vi "01_Main.vi"() -> ()   [LabVIEW 2023]
doc: "This VI shows how to setup and execute a measurement without any user input."
panel:
  out "N":i32=-1
  out "size(s)":i32[](array[numeric])
  in  "Fahrprofil Datei":path
  out "IP-Adresse Antrieb":string="192.168.10.5"
  in  "BETRIEBSART ANTRIEB":bool
  out "Digital Antrieb":dbl
  out "Drehmoment Antrieb":dbl
  out "Status/Fehler Antrieb":dbl
  out "Istgeschwindigkeit Antrieb":dbl
  in  "Digital Antrieb":dbl
  in  "Deceleration Antrieb":dbl
  in  "Acceleration Antrieb":dbl
  in  "Speed Antrieb":dbl
  out "IP-Adresse Last":string
  out "Digital":dbl
  out "Drehmoment":dbl
  out "Status/Fehler":dbl
  out "Istgeschwindigkeit":dbl
  in  "Digital A":dbl
  in  "Deceleration":dbl
  in  "Acceleration":dbl
  in  "Speed":dbl
  out "Reserviert":bool
  out "SWES inaktiv":bool
  out "Geschwindigkeit erreicht":bool
  out "Warnung":bool
  out "Fehler":bool
  out "in Position":bool
  out "Relativposition übernommen":bool
  out "Motor dreht":bool
  out "Bremse geöffnet":bool
  out "Endstufenfreigabe":bool
  out "STO inaktiv":bool
  out "Betriebsbereit":bool
  out "Reserviert 8":bool
  out "SWES inaktiv 2":bool
  out "Geschwindigkeit erreicht 2":bool
  out "Warnung 2":bool
  out "Fehler 2":bool
  out "in Position 2":bool
  out "Relativposition übernommen 2":bool
  out "Motor dreht 2":bool
  out "Bremse geöffnet 2":bool
  out "Endstufenfreigabe 2":bool
  out "STO inaktiv 2":bool
  out "Betriebsbereit 2":bool
  in  "Reserviert 9":bool
  in  "Reservier 2":bool
  in  "Reserviert 10":bool
  in  "Reserviert 11":bool
  in  "Reserviert 12":bool
  in  "Reserviert 13":bool
  in  "Reserviert 14":bool
  in  "Reserviert 2":bool
  in  "Reservier":bool
  in  "Reserviert 3":bool
  in  "Reserviert 4":bool
  in  "Reserviert 5":bool
  in  "Reserviert 6":bool
  in  "Reserviert 7":bool
  in  "Bedienelemente - Lastmotor":enum32{"Standard", "Versteckt"}(tab)
  in  "Enable/EmergencyStop Antrieb":bool
  in  "Fehler_Reset Antrieb":bool
  in  "Antriebsmotor Start":bool
  in  "Enable/ApplicationStop Antrieb":bool=TRUE
  in  "Inhibit L":bool
  in  "Standby Antrieb":bool
  in  "Handshake Antrieb":bool
  in  "AS2 aktivieren Antrieb":bool
  in  "Bremse öffnen Antrieb":bool
  out "Standby aktiv 2":bool
  out "AS2 aktiv 2":bool
  out "Handshake 3":bool
  out "referenziert 2":bool
  in  "Bedienelemente - Antriebsmotor":enum32{"Standard", "Versteckt"}(tab)
  in  "Enable/EmergencyStop":bool
  in  "Enable/ApplicationStop":bool=TRUE
  in  "Fehler_Reset":bool
  in  "Lastmotor Start":bool
  in  "Inhibit":bool
  in  "Standby":bool
  in  "Handshake 2":bool
  in  "AS2 aktivieren":bool
  in  "Bremse öffnen":bool
  out "AS2 aktiv":bool
  out "Handshake":bool
  out "Standby aktiv":bool
  out "referenziert":bool
  out "Numeric":i32
  out "VI wird beendet":string
  in  "VI-Stopp":bool
  out "Diagram 2":waveform(dbl)(graph)
  in  "Kanal 2":i32=2 min=1 max=4 step=1
  in  "Kanal":i32=1 min=1 max=4 step=1
  in  "Datei-Pfad":path
  out "Diagram":waveform(dbl)(graph)
  in  "Messung":bool=TRUE
  out "HBM Driver\nLicense is valid":bool
  # "Im Handbetrieb im Feld \"Speed\" die Soll-Geschwindigkeit vorgeben. Nach Betätigung des Start-Knopfes läuft der Motor an. \n\nFür den Antrieb ist das Laden von Fahrprofilen möglich. Dazu Fahrprofil Datei auswählen, START-Knopf drücken und dann BETRIEBSART ANTRIEB auf \"Fahrprofile laden\" schalten."
  # "Handbetrieb"
  # "Fahrprofil laden"
  # "Manuelle Ansteuerung des Last-Motors"
  # "Manuelle Ansteuerung des Antrieb-Motors"
  # "Datenaquise mit dem HBM Messverstärker"
  # "Messung mit START starten.\n\nWenn die Messdaten gespeichert werden sollen, muss vor \ndem Starten der Messung ein gültiger Dateipfad angegeben werden."
  # "Datenaufzeichnung"
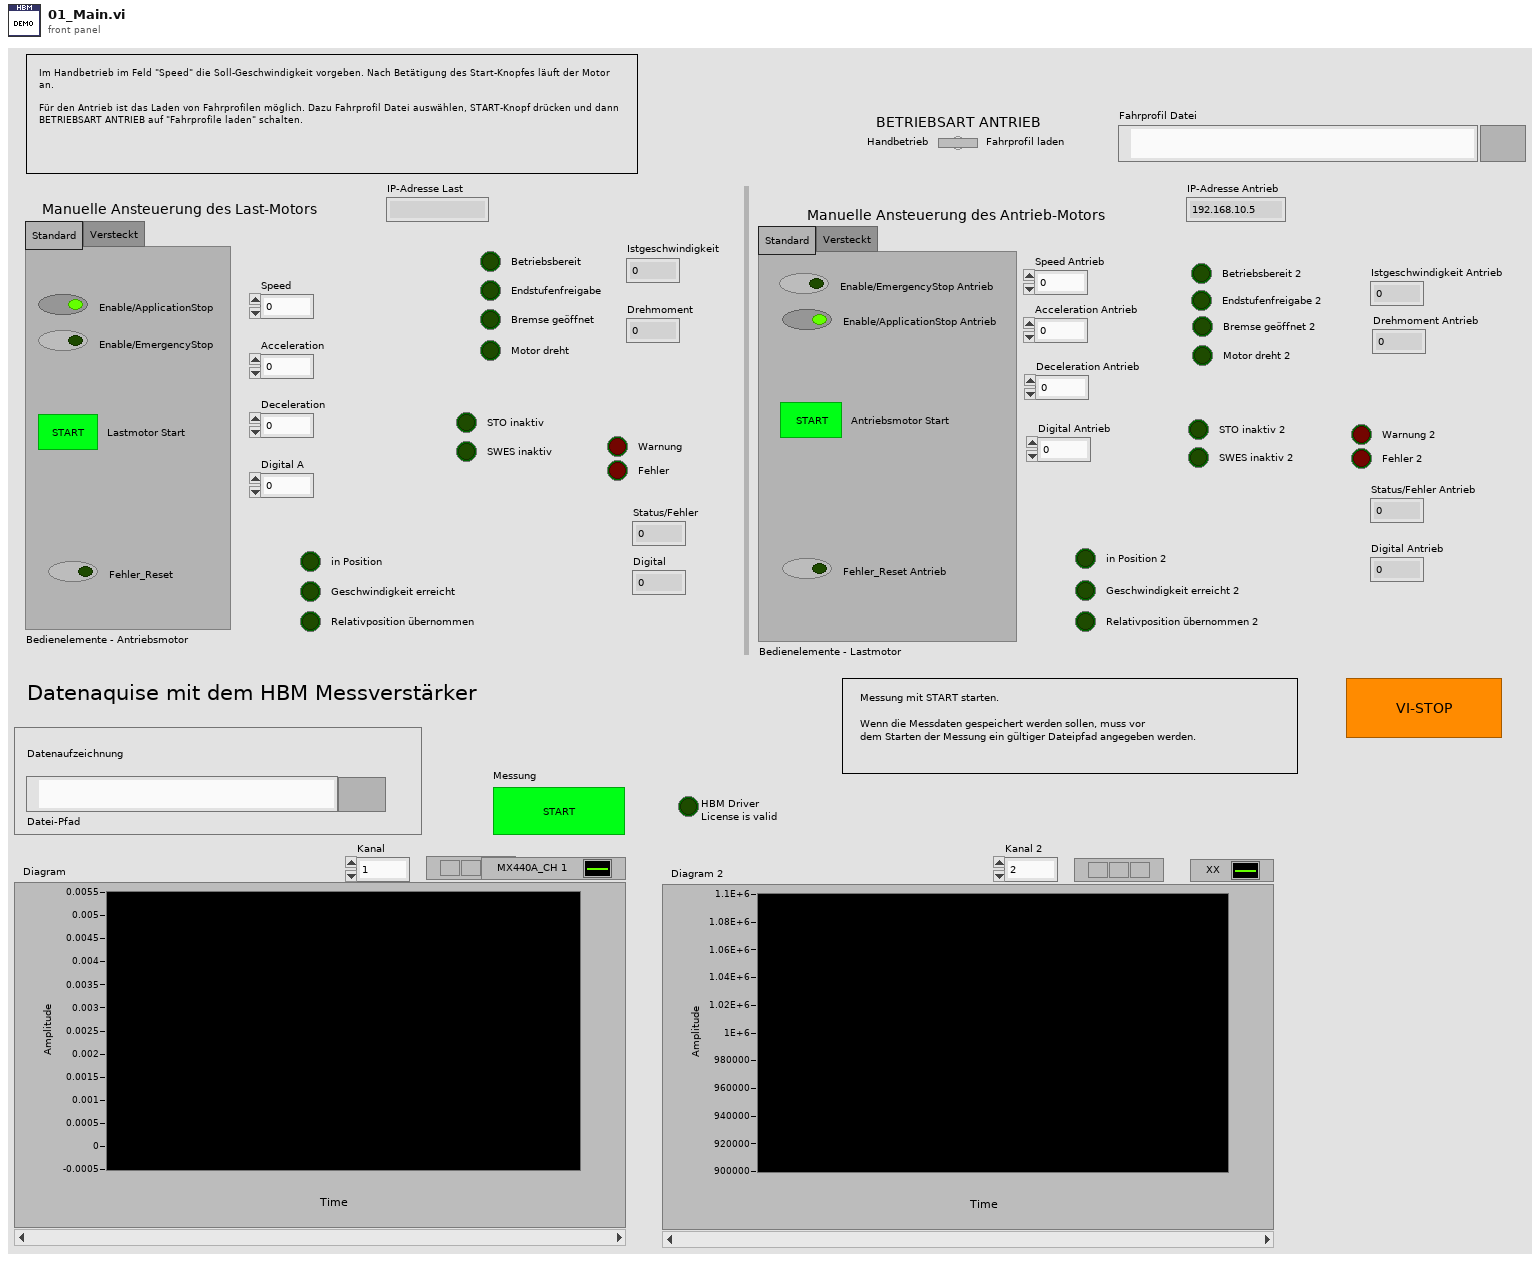
[diagram p1: front panel]
types:
  T1 = cluster{"Devices":refnum<k24>[], "Signals":refnum<k24>[]}
  T2 = enum16{"open", "replace", "create", "open or create", "replace or create", "replace or create with confirmation"}
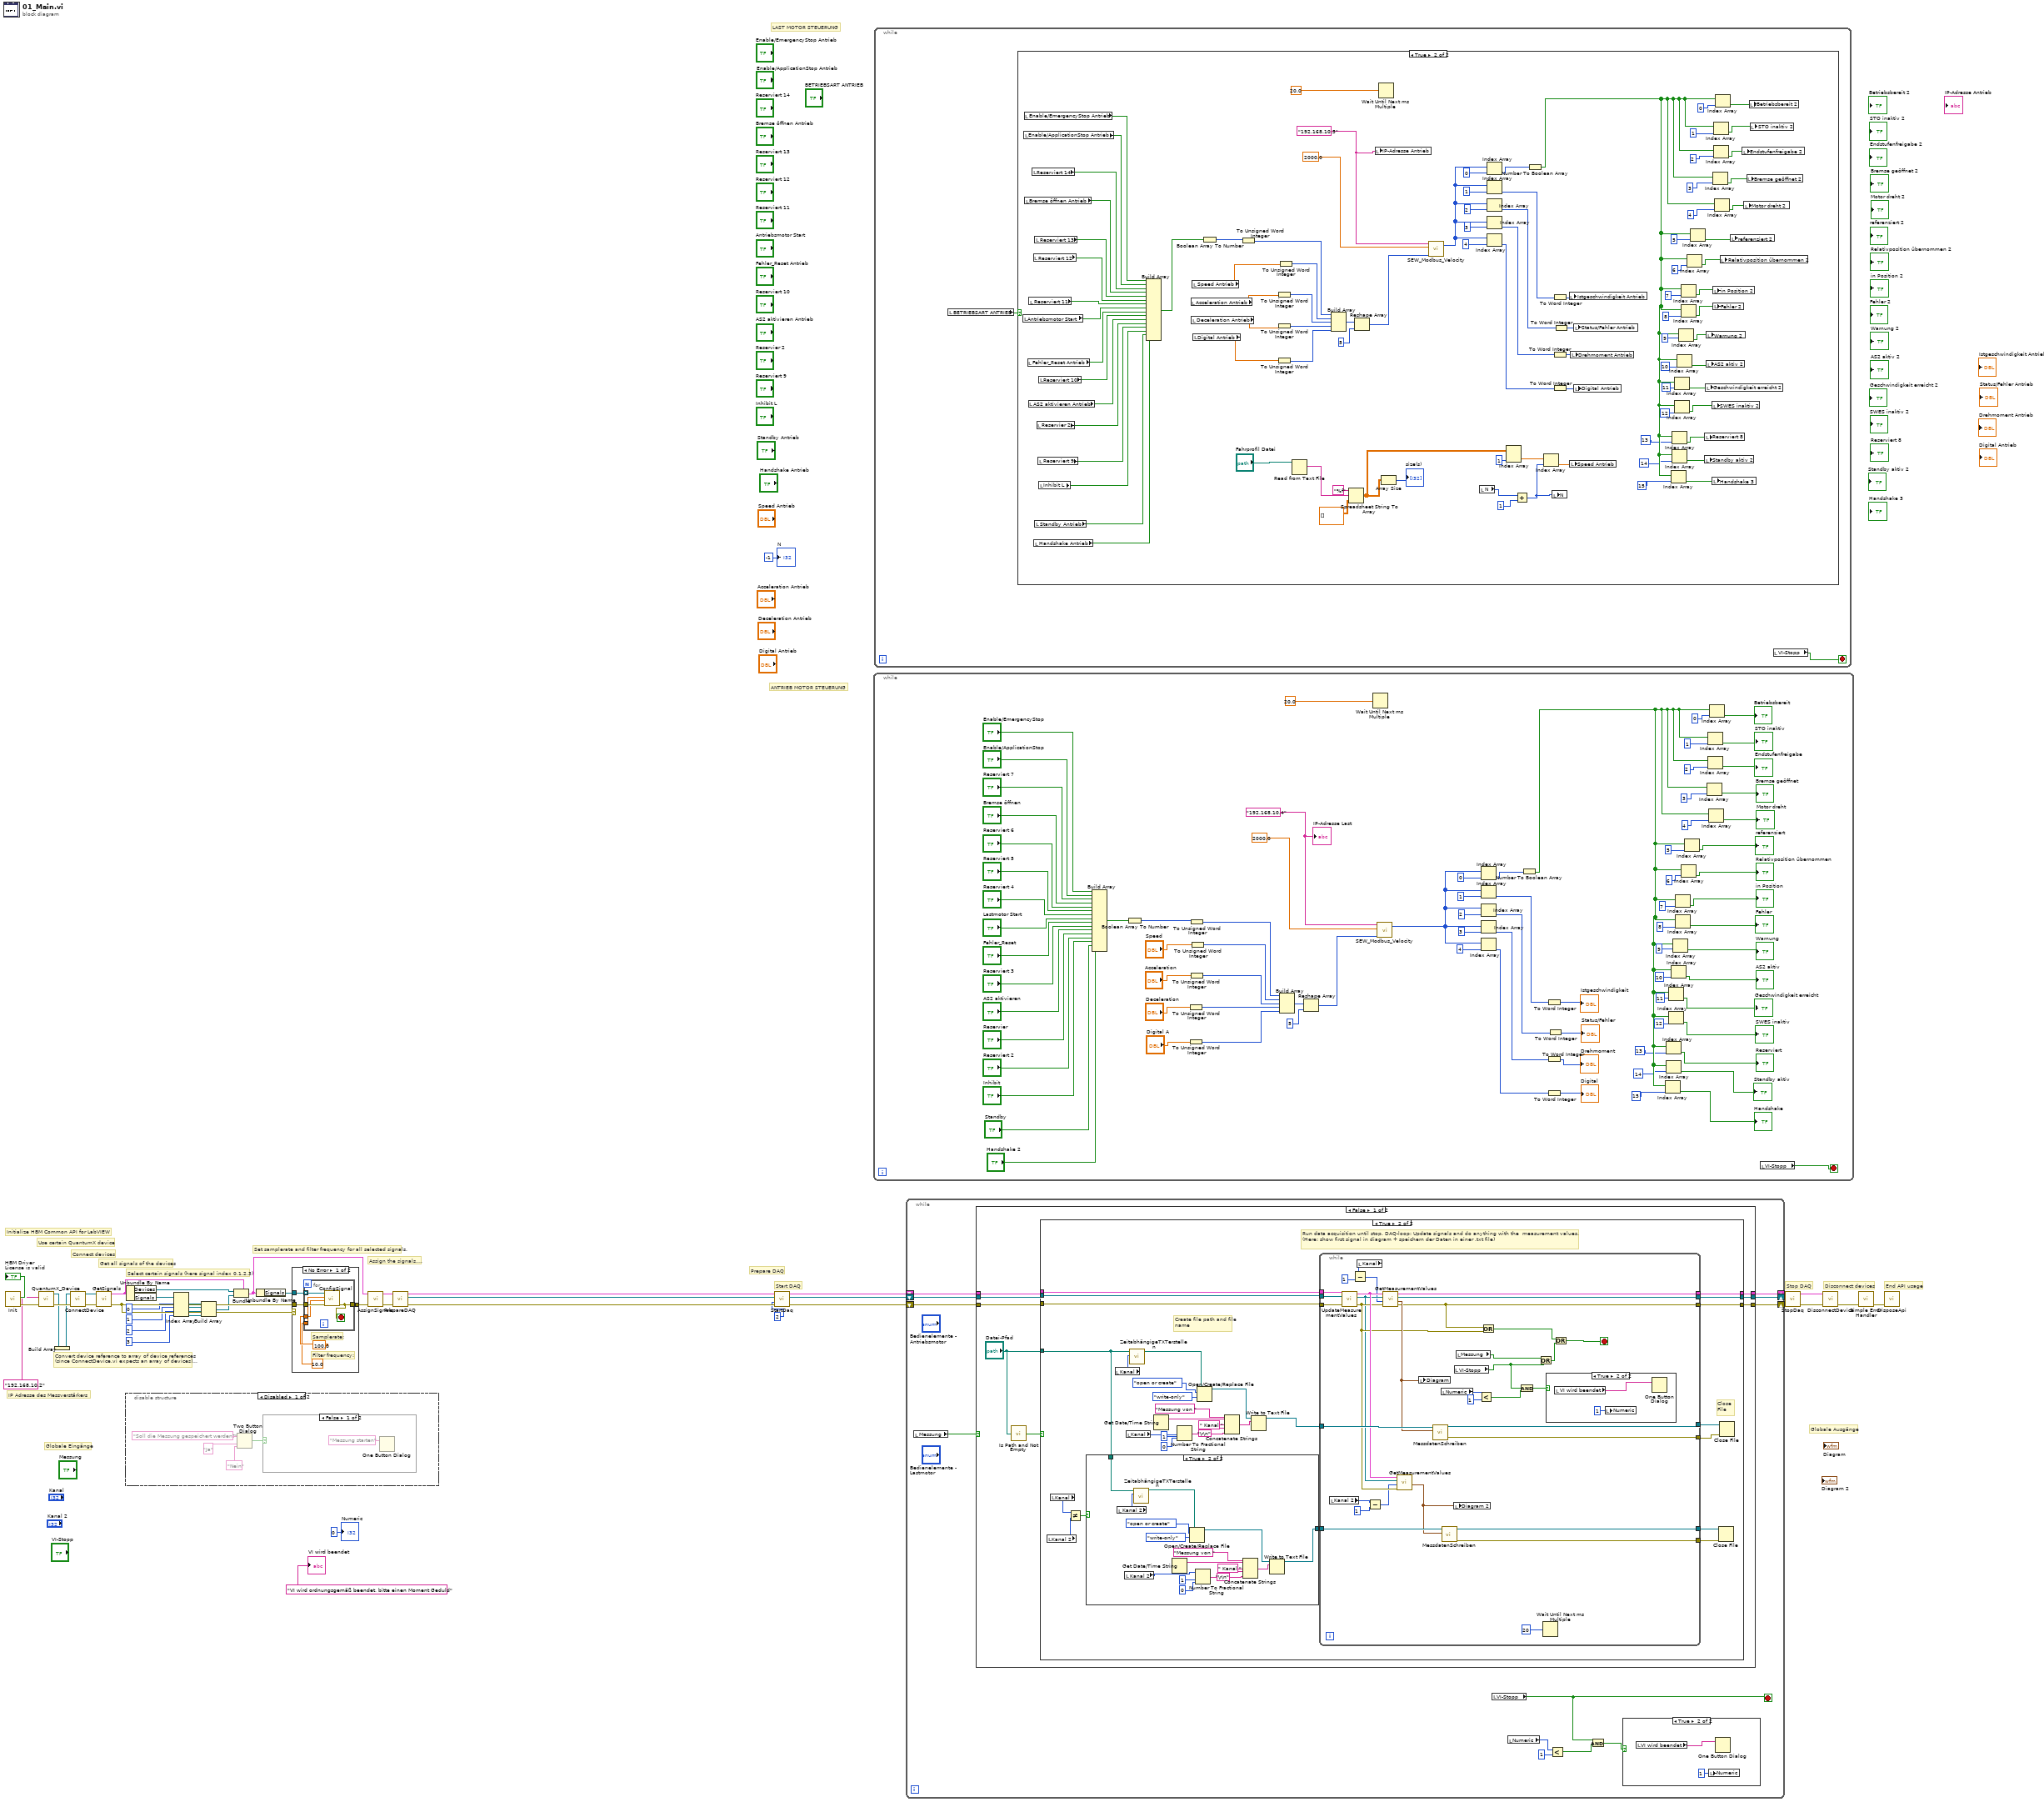
[diagram p0: block diagram]
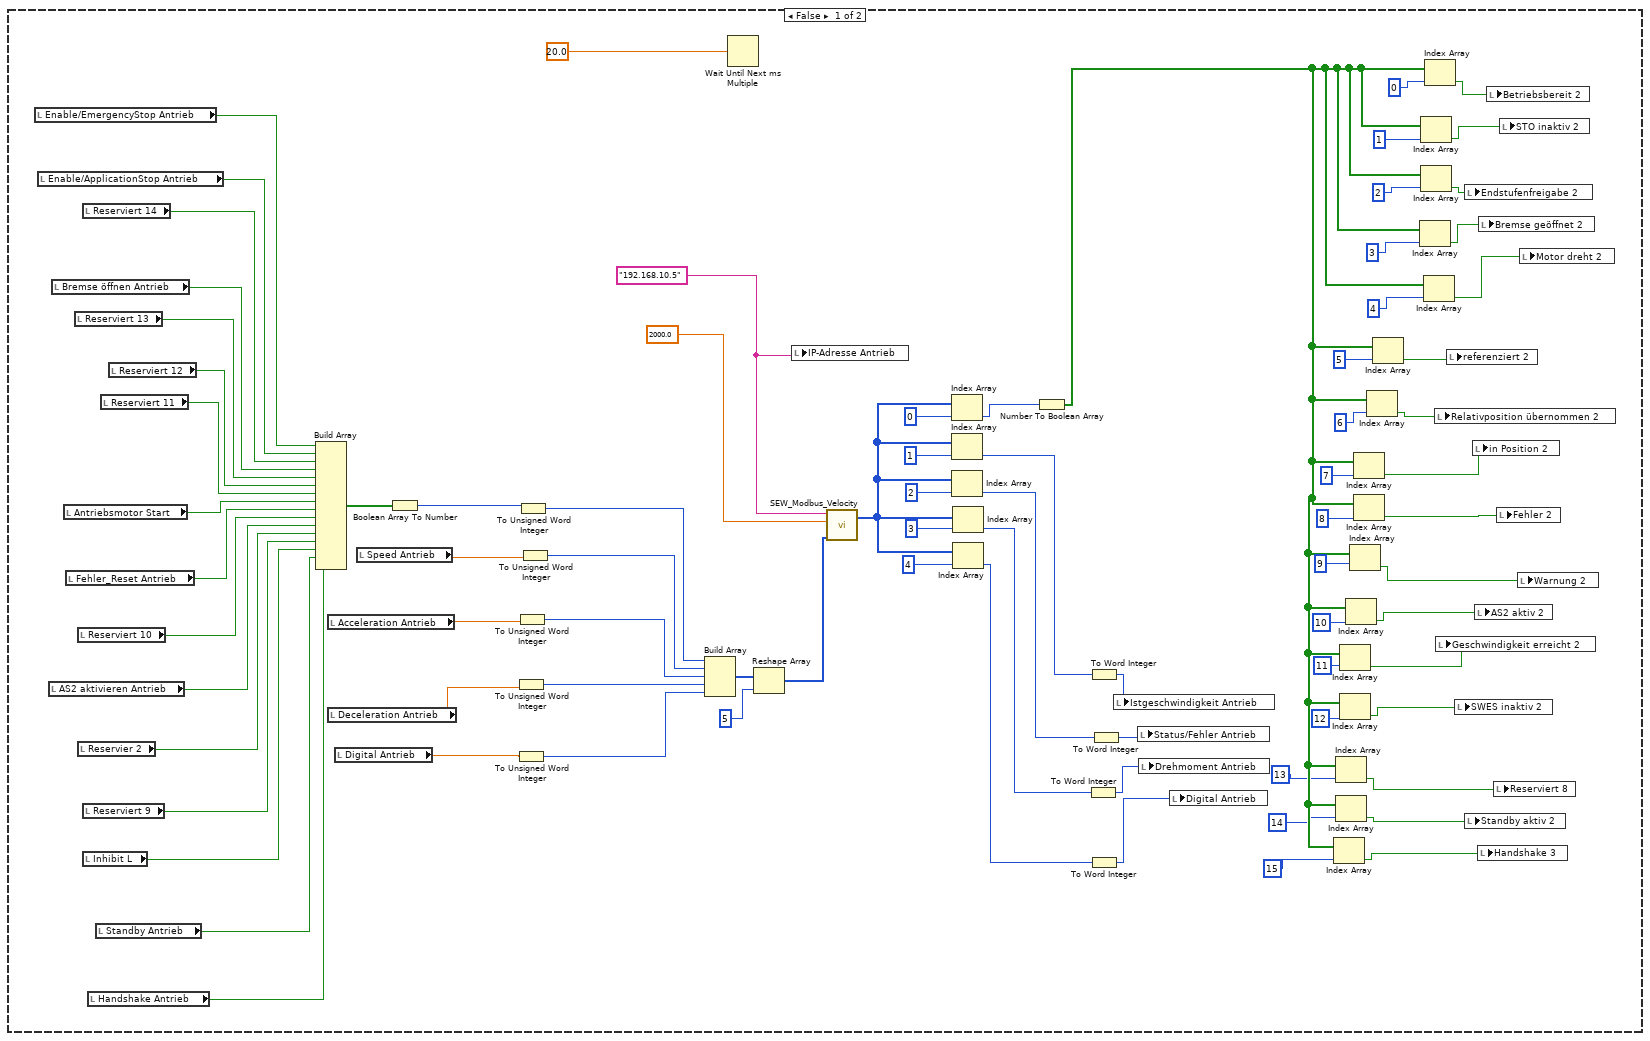
[diagram p2: hidden frame]
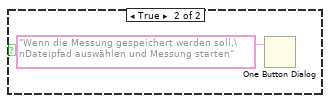
[diagram p3: hidden frame]
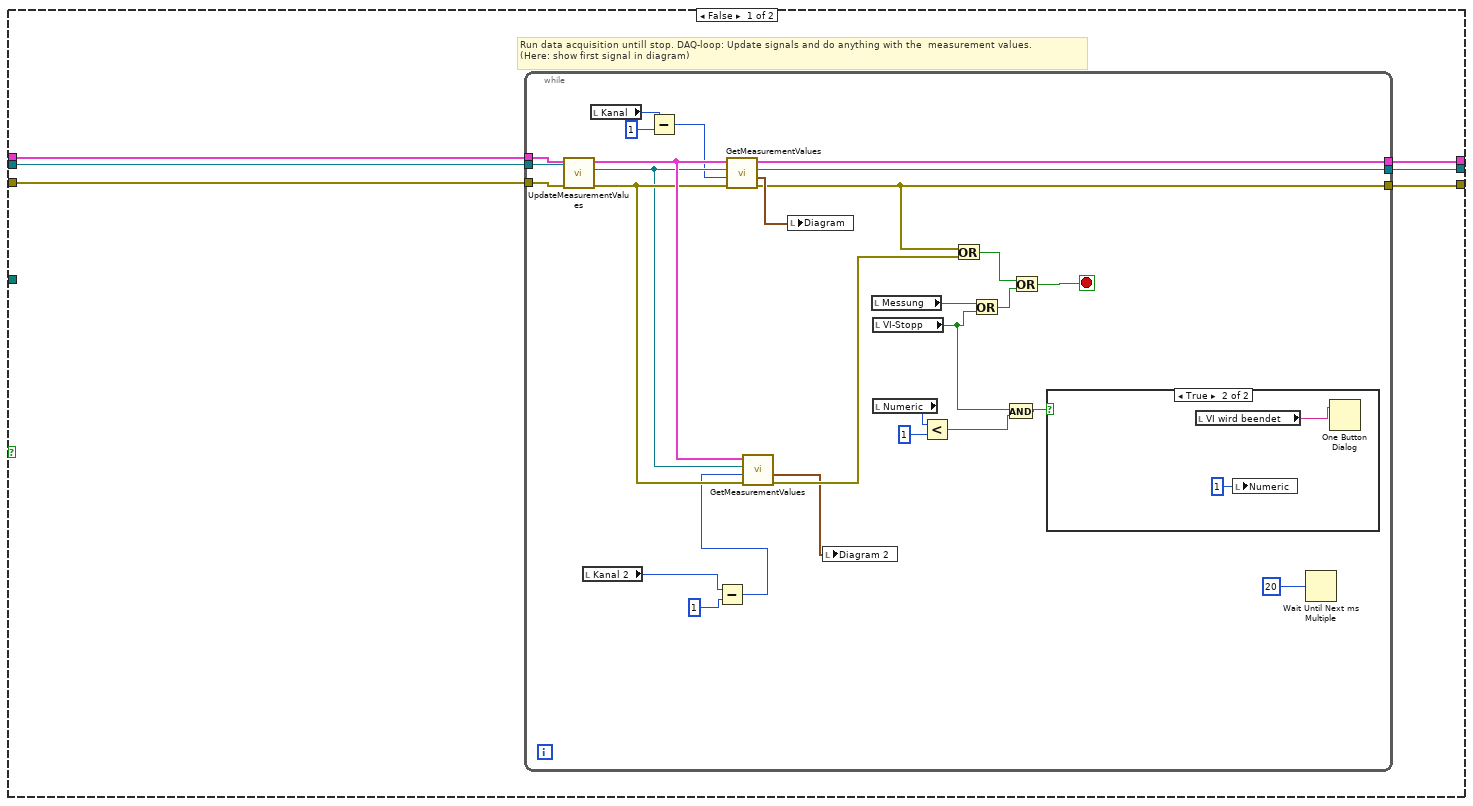
[diagram p6: hidden frame]
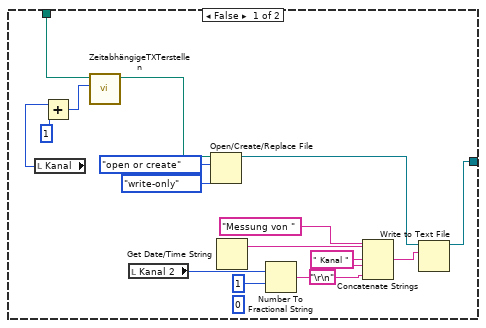
[diagram p8: hidden frame]
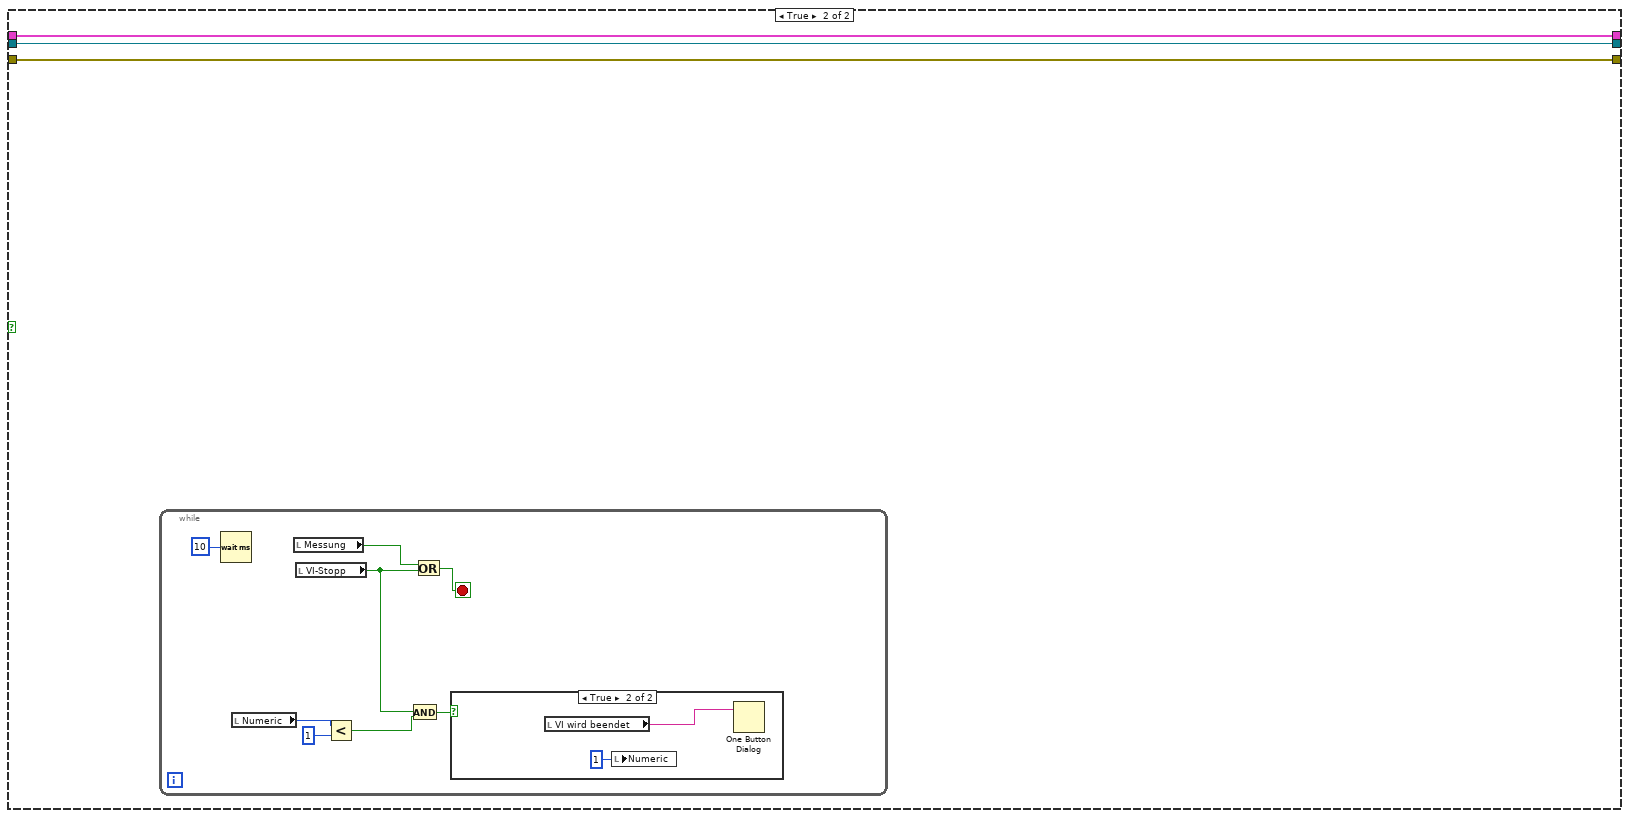
[diagram p10: hidden frame]
diagram:
  # "ANTRIEB MOTOR STEUERUNG"
  # "LAST MOTOR STEUERUNG"
  # "Globale Ausgänge"
  # "Globale Eingänge"
  # "IP Adresse des Messverstärkers"
  # "Convert device reference to array of device references\n(since ConnectDevice.vi expects an array of devices)..."
  # "Disconnect devices"
  # "Set samplerate and filter frequency for all selected signals."
  # "Initialize HBM Common API for LabVIEW"
  # "End API usage"
  # "Stop DAQ"
  # "Start DAQ"
  # "Prepare DAQ"
  # "Select certain signals (here signal index 0,1,2,3)"
  # "Get all signals of the devices"
  # "Connect devices"
  # "Use certain QuantumX device"
  # "Assign the signals...."
  n1 = call <userlib>:"Init.vi"() -> ("LicenseIsValid"=→"HBM Driver\nLicense is valid":bool, "Error out"=w13:errorcluster)  [unwired: 8 in, 1 out]
  n2 = call <userlib>:"QuantumX_Device.vi"("Error in"=w13, "IPAddress"="192.168.10.2" ("IPAddress of QuantumX device")) -> ("Error out"=w14:errorcluster, "Device"=w11:refnum<k24>)  [unwired: 6 in]
  n3 = Build Array(w11) -> (w10:refnum<k24>[])
  n4 = call <userlib>:"ConnectDevice.vi"("Error in"=w14, "Devices"=w10) -> ("Error out"=w36:errorcluster, "Devices"=w35:refnum<k24>[])  [unwired: 7 in, 1 out]
  n5 = call <userlib>:"GetSignals.vi"("Error in"=w36, "Devices"=w35) -> ("Error out"=w30:errorcluster, "DevicesAndSignals"=w31:T1)  [unwired: 8 in]
  n6 = disable-structure shown="Disabled" {
    frame Disabled {
      n7 = Two Button Dialog(message="Soll die Messung gespeichert werden?", 1:"Nein" ("F button name (\"Cancel\")"), 2:"Ja" ("T button name (\"OK\")")) -> (T button?=w47:bool)
      n8 = case shown="False" w47 {
        frame False {
          n9 = One Button Dialog(message="Messung starten") -> ()  [unwired: 1 in, 1 out]
        }
        frame True {
          n10 = One Button Dialog(message="Wenn die Messung gespeichert werden soll,\nDateipfad auswählen und Messung starten") -> ()  [unwired: 1 in, 1 out]
        }
      }
    }
    frame Enabled {
    }
  }
  n11 = Unbundle By Name(w31) -> ("Devices"=w24:refnum<k24>[], "Signals"=w28:refnum<k24>[])
  n12 = Index Array(array=w28, index #1=0 ("Index"), index #2=1 ("Index"), index #3=2 ("Index"), index #4=3 ("Index")) -> (element #1=w27:refnum<k24>, element #2=w26:refnum<k24>, element #3=w19:refnum<k24>, element #4=w18:refnum<k24>)
  n13 = Build Array(w27, w26, w19, w18) -> (w25:refnum<k24>[])
  n14 = Bundle(cluster=w31, "Devices"=w24, "Signals"=w25) -> (w32:T1)
  n15 = Unbundle By Name(w32) -> ("Signals"=w43:refnum<k24>[])
  n16 = case shown="No Error" w30 {
    tunnel: w30 -> [w54 w60]
    tunnel: w43 -> [w53 _]
    tunnel: [w52 w60] -> w42
    frame No Error {
      # "Filter frequency:"
      # "Samplerate:"
      n17 = for {
        tunnel: w54 -> [w59]
        tunnel: 100.0 ("SampleRate") -> [w58]
        tunnel: 10.0 ("FilterFrequency") -> [w57]
        tunnel: w53 -> [w56] mode=indexing
        tunnel: [w55] -> w52
        stop <- w55 stop-if-true
        n18 = call <userlib>:"ConfigSignal.vi"("Error in"=w59, "SampleRate"=w58, "FilterFrequency"=w57, "Signal"=w56) -> ("Error out"=w55:errorcluster)  [unwired: 7 in]
      }
    }
    frame Error {
    }
  }
  n19 = call <userlib>:"AssignSignals.vi"("Error in"=w42, "DevicesAndSignals"=w32) -> ("Error out"=w40:errorcluster, "DevicesAndSignals"=w41:T1)  [unwired: 8 in]
  n20 = call <userlib>:"PrepareDAQ.vi"("Error in"=w40, "DevicesAndSignals"=w41) -> ("Error out"=w37:errorcluster, "DaqMeasurement"=w38:refnum<k24>, "DevicesAndSignals"=w39:T1)  [unwired: 7 in]
  n21 = call <userlib>:"StartDaq.vi"("DevicesAndSignals"=w39, "DaqMeasurement"=w38, "AcquisitionMode"=2, "Error in"=w37) -> ("DevicesAndSignals"=w6:T1, "DaqMeasurement"=w5:refnum<k24>, "Error out"=w4:errorcluster)  [unwired: 7 in, 2 out]
  n22 = while {
    stop <- w102 stop-if-true
    w101 = "192.168.10.4"
    n23 = Build Array("Enable/EmergencyStop", "Enable/ApplicationStop", "Reserviert 7", "Bremse öffnen", "Reserviert 6", "Reserviert 5", "Reserviert 4", "Lastmotor Start", "Fehler_Reset", "Reserviert 3", "AS2 aktivieren", "Reservier", "Reserviert 2", "Inhibit", "Standby", "Handshake 2") -> (w135:bool[])
    n24 = Boolean Array To Number(Boolean array=w135) -> (number=w136:u32)
    n25 = To Unsigned Word Integer(number="Deceleration") -> (unsigned 16bit integer=w139:u16)
    n26 = To Unsigned Word Integer(number="Digital A") -> (unsigned 16bit integer=w140:u16)
    n27 = To Unsigned Word Integer(number="Acceleration") -> (unsigned 16bit integer=w138:u16)
    n28 = To Unsigned Word Integer(number=w136) -> (unsigned 16bit integer=w137:u16)
    n29 = To Unsigned Word Integer(number="Speed") -> (unsigned 16bit integer=w141:u16)
    n30 = Build Array(w137, w141, w138, w139, w140) -> (w142:u16[])
    n31 = Reshape Array(w142, 5) -> (w132:u16[])
    n32 = Wait Until Next ms Multiple(millisecond multiple=20.0 ("Update(ms)")) -> ()  [unwired: 1 out]
    n33 = call "SEW_Modbus_Velocity.vi"("Remote IP Address"=w101, "Timeout [ms]"=2000.0 ("Timeout (ms)"), "Output (Write Multiple Register) 2"=w132) -> ("Input (Read Holding Register) 2"=w130:u16[])  [unwired: 3 in]
    n34 = Index Array(array=w130, index=0) -> (element=w120:u16)
    n35 = Index Array(array=w130, index=1) -> (element=w121:u16)
    n36 = Index Array(array=w130, index=2) -> (element=w122:u16)
    n37 = Index Array(array=w130, index=3) -> (element=w123:u16)
    n38 = Index Array(array=w130, index=4) -> (element=w124:u16)
    n39 = Number To Boolean Array(number=w120) -> (Boolean array=w119:bool[])
    n40 = To Word Integer(number=w123) -> (16bit integer=→"Drehmoment":i16)
    n41 = To Word Integer(number=w121) -> (16bit integer=→"Istgeschwindigkeit":i16)
    n42 = To Word Integer(number=w124) -> (16bit integer=→"Digital":i16)
    n43 = To Word Integer(number=w122) -> (16bit integer=→"Status/Fehler":i16)
    n44 = Index Array(array=w119, index=15) -> (element=→"Handshake":bool)
    n45 = Index Array(array=w119, index=13) -> (element=→"Reserviert":bool)
    n46 = Index Array(array=w119, index=14) -> (element=→"Standby aktiv":bool)
    n47 = Index Array(array=w119, index=11) -> (element=→"Geschwindigkeit erreicht":bool)
    n48 = Index Array(array=w119, index=12) -> (element=→"SWES inaktiv":bool)
    n49 = Index Array(array=w119, index=10) -> (element=→"AS2 aktiv":bool)
    n50 = Index Array(array=w119, index=9) -> (element=→"Warnung":bool)
    n51 = Index Array(array=w119, index=7) -> (element=→"in Position":bool)
    n52 = Index Array(array=w119, index=8) -> (element=→"Fehler":bool)
    n53 = Index Array(array=w119, index=6) -> (element=→"Relativposition übernommen":bool)
    n54 = Index Array(array=w119, index=5) -> (element=→"referenziert":bool)
    n55 = Index Array(array=w119, index=3) -> (element=→"Bremse geöffnet":bool)
    n56 = Index Array(array=w119, index=1) -> (element=→"STO inaktiv":bool)
    n57 = Index Array(array=w119, index=2) -> (element=→"Endstufenfreigabe":bool)
    n58 = Index Array(array=w119, index=4) -> (element=→"Motor dreht":bool)
    n59 = Index Array(array=w119, index=0) -> (element=→"Betriebsbereit":bool)
    n60 = local read "VI-Stopp"() -> (w102:bool)
    "IP-Adresse Last" <- w101
  }
  n61 = while {
    stop <- w143 stop-if-true
    n62 = local read "BETRIEBSART ANTRIEB"() -> (w144:bool)
    n63 = case shown="True" w144 {
      frame False {
        w145 = "192.168.10.5"
        n64 = local read "Enable/EmergencyStop Antrieb"() -> (w169:bool)
        n65 = local read "Enable/ApplicationStop Antrieb"() -> (w168:bool)
        n66 = local read "AS2 aktivieren Antrieb"() -> (w158:bool)
        n67 = local read "Bremse öffnen Antrieb"() -> (w166:bool)
        n68 = local read "Antriebsmotor Start"() -> (w156:bool)
        n69 = local read "Fehler_Reset Antrieb"() -> (w157:bool)
        n70 = local read "Reserviert 13"() -> (w165:bool)
        n71 = local read "Reserviert 10"() -> (w160:bool)
        n72 = local read "Reservier 2"() -> (w159:bool)
        n73 = local read "Reserviert 14"() -> (w167:bool)
        n74 = local read "Reserviert 9"() -> (w161:bool)
        n75 = local read "Inhibit L"() -> (w162:bool)
        n76 = local read "Handshake Antrieb"() -> (w164:bool)
        n77 = local read "Standby Antrieb"() -> (w163:bool)
        n78 = local read "Reserviert 11"() -> (w155:bool)
        n79 = local read "Reserviert 12"() -> (w154:bool)
        n80 = Build Array(w169, w168, w167, w166, w165, w154, w155, w156, w157, w160, w158, w159, w161, w162, w163, w164) -> (w218:bool[])
        n81 = local read "Acceleration Antrieb"() -> (w148:dbl)
        n82 = local read "Deceleration Antrieb"() -> (w147:dbl)
        n83 = local read "Digital Antrieb"() -> (w146:dbl)
        n84 = local read "Speed Antrieb"() -> (w149:dbl)
        n85 = Boolean Array To Number(Boolean array=w218) -> (number=w219:u32)
        n86 = To Unsigned Word Integer(number=w147) -> (unsigned 16bit integer=w222:u16)
        n87 = To Unsigned Word Integer(number=w146) -> (unsigned 16bit integer=w223:u16)
        n88 = To Unsigned Word Integer(number=w148) -> (unsigned 16bit integer=w221:u16)
        n89 = To Unsigned Word Integer(number=w219) -> (unsigned 16bit integer=w220:u16)
        n90 = To Unsigned Word Integer(number=w149) -> (unsigned 16bit integer=w224:u16)
        n91 = Build Array(w220, w224, w221, w222, w223) -> (w225:u16[])
        n92 = Wait Until Next ms Multiple(millisecond multiple=20.0 ("Update(ms)")) -> ()  [unwired: 1 out]
        n93 = Reshape Array(w225, 5) -> (w215:u16[])
        n94 = local write "IP-Adresse Antrieb"(w145) -> ()
        n95 = call "SEW_Modbus_Velocity.vi"("Remote IP Address"=w145, "Timeout [ms]"=2000.0 ("Timeout (ms)"), "Output (Write Multiple Register) 2"=w215) -> ("Input (Read Holding Register) 2"=w213:u16[])  [unwired: 3 in]
        n96 = Index Array(array=w213, index=0) -> (element=w203:u16)
        n97 = Index Array(array=w213, index=1) -> (element=w204:u16)
        n98 = Index Array(array=w213, index=2) -> (element=w205:u16)
        n99 = Index Array(array=w213, index=3) -> (element=w206:u16)
        n100 = Index Array(array=w213, index=4) -> (element=w207:u16)
        n101 = Number To Boolean Array(number=w203) -> (Boolean array=w202:bool[])
        n102 = To Word Integer(number=w206) -> (16bit integer=w151:i16)
        n103 = To Word Integer(number=w204) -> (16bit integer=w153:i16)
        n104 = To Word Integer(number=w207) -> (16bit integer=w150:i16)
        n105 = To Word Integer(number=w205) -> (16bit integer=w152:i16)
        n106 = local write "Istgeschwindigkeit Antrieb"(w153) -> ()
        n107 = local write "Status/Fehler Antrieb"(w152) -> ()
        n108 = local write "Drehmoment Antrieb"(w151) -> ()
        n109 = local write "Digital Antrieb"(w150) -> ()
        n110 = Index Array(array=w202, index=15) -> (element=w170:bool)
        n111 = Index Array(array=w202, index=13) -> (element=w172:bool)
        n112 = Index Array(array=w202, index=14) -> (element=w171:bool)
        n113 = Index Array(array=w202, index=11) -> (element=w174:bool)
        n114 = Index Array(array=w202, index=12) -> (element=w173:bool)
        n115 = Index Array(array=w202, index=10) -> (element=w175:bool)
        n116 = Index Array(array=w202, index=9) -> (element=w176:bool)
        n117 = Index Array(array=w202, index=7) -> (element=w178:bool)
        n118 = Index Array(array=w202, index=8) -> (element=w177:bool)
        n119 = Index Array(array=w202, index=6) -> (element=w179:bool)
        n120 = Index Array(array=w202, index=5) -> (element=w180:bool)
        n121 = Index Array(array=w202, index=3) -> (element=w182:bool)
        n122 = Index Array(array=w202, index=1) -> (element=w184:bool)
        n123 = Index Array(array=w202, index=2) -> (element=w183:bool)
        n124 = Index Array(array=w202, index=4) -> (element=w181:bool)
        n125 = Index Array(array=w202, index=0) -> (element=w185:bool)
        n126 = local write "Relativposition übernommen 2"(w179) -> ()
        n127 = local write "Geschwindigkeit erreicht 2"(w174) -> ()
        n128 = local write "referenziert 2"(w180) -> ()
        n129 = local write "SWES inaktiv 2"(w173) -> ()
        n130 = local write "Endstufenfreigabe 2"(w183) -> ()
        n131 = local write "Standby aktiv 2"(w171) -> ()
        n132 = local write "in Position 2"(w178) -> ()
        n133 = local write "AS2 aktiv 2"(w175) -> ()
        n134 = local write "Handshake 3"(w170) -> ()
        n135 = local write "Bremse geöffnet 2"(w182) -> ()
        n136 = local write "Betriebsbereit 2"(w185) -> ()
        n137 = local write "Reserviert 8"(w172) -> ()
        n138 = local write "Fehler 2"(w177) -> ()
        n139 = local write "STO inaktiv 2"(w184) -> ()
        n140 = local write "Warnung 2"(w176) -> ()
        n141 = local write "Motor dreht 2"(w181) -> ()
      }
      frame True {
        w238 = "192.168.10.5"
        n142 = local read "Antriebsmotor Start"() -> (w266:bool)
        n143 = local read "Enable/ApplicationStop Antrieb"() -> (w260:bool)
        n144 = local read "Enable/EmergencyStop Antrieb"() -> (w259:bool)
        n145 = local read "Bremse öffnen Antrieb"() -> (w262:bool)
        n146 = local read "Fehler_Reset Antrieb"() -> (w267:bool)
        n147 = local read "AS2 aktivieren Antrieb"() -> (w269:bool)
        n148 = local read "Reserviert 11"() -> (w265:bool)
        n149 = local read "Reserviert 14"() -> (w261:bool)
        n150 = local read "Reserviert 12"() -> (w264:bool)
        n151 = local read "Handshake Antrieb"() -> (w274:bool)
        n152 = local read "Reserviert 13"() -> (w263:bool)
        n153 = local read "Standby Antrieb"() -> (w273:bool)
        n154 = local read "Reservier 2"() -> (w270:bool)
        n155 = local read "Reserviert 9"() -> (w271:bool)
        n156 = local read "Reserviert 10"() -> (w268:bool)
        n157 = local read "Inhibit L"() -> (w272:bool)
        n158 = Build Array(w259, w260, w261, w262, w263, w264, w265, w266, w267, w268, w269, w270, w271, w272, w273, w274) -> (w311:bool[])
        n159 = local read "Acceleration Antrieb"() -> (w277:dbl)
        n160 = local read "Deceleration Antrieb"() -> (w276:dbl)
        n161 = local read "Speed Antrieb"() -> (w278:dbl)
        n162 = local read "Digital Antrieb"() -> (w275:dbl)
        n163 = Boolean Array To Number(Boolean array=w311) -> (number=w312:u32)
        n164 = To Unsigned Word Integer(number=w312) -> (unsigned 16bit integer=w313:u16)
        n165 = To Unsigned Word Integer(number=w276) -> (unsigned 16bit integer=w315:u16)
        n166 = To Unsigned Word Integer(number=w275) -> (unsigned 16bit integer=w316:u16)
        n167 = To Unsigned Word Integer(number=w277) -> (unsigned 16bit integer=w314:u16)
        n168 = To Unsigned Word Integer(number=w278) -> (unsigned 16bit integer=w317:u16)
        n169 = Read from Text File(file (use dialog)="Fahrprofil Datei") -> (text=w235:string)  [unwired: 2 in, 4 out]
        n170 = Build Array(w313, w317, w314, w315, w316) -> (w318:u16[])
        n171 = Spreadsheet String To Array(format string="%f", spreadsheet string=w235, array type (2D Dbl)=dbl[][] []) -> (array=w230:dbl[][])  [unwired: 1 in]
        n172 = Reshape Array(w318, 5) -> (w308:u16[])
        n173 = local write "IP-Adresse Antrieb"(w238) -> ()
        n174 = Wait Until Next ms Multiple(millisecond multiple=20.0 ("Update(ms)")) -> ()  [unwired: 1 out]
        n175 = Array Size(array=w230) -> (size(s)=→"size(s)":i32[])
        n176 = call "SEW_Modbus_Velocity.vi"("Remote IP Address"=w238, "Timeout [ms]"=2000.0 ("Timeout (ms)"), "Output (Write Multiple Register) 2"=w308) -> ("Input (Read Holding Register) 2"=w306:u16[])  [unwired: 3 in]
        n177 = local read "N"() -> (w228:i32)
        n178 = Index Array(array=w306, index=0) -> (element=w296:u16)
        n179 = Index Array(array=w306, index=1) -> (element=w297:u16)
        n180 = Index Array(array=w306, index=2) -> (element=w298:u16)
        n181 = Index Array(array=w306, index=3) -> (element=w299:u16)
        n182 = Index Array(array=w306, index=4) -> (element=w300:u16)
        n183 = Index Array(array=w230, index (col)=1 ("disabled index (col)")) -> (element=w237:dbl[])  [unwired: 1 in]
        n184 = Add(x=w228, y=1) -> (x+y=w226:i32)
        n185 = Number To Boolean Array(number=w296) -> (Boolean array=w295:bool[])
        n186 = Index Array(array=w237, index=w226) -> (element=w229:dbl)
        n187 = To Word Integer(number=w299) -> (16bit integer=w256:i16)
        n188 = local write "N"(w226) -> ()
        n189 = To Word Integer(number=w297) -> (16bit integer=w258:i16)
        n190 = To Word Integer(number=w300) -> (16bit integer=w255:i16)
        n191 = To Word Integer(number=w298) -> (16bit integer=w257:i16)
        n192 = local write "Istgeschwindigkeit Antrieb"(w258) -> ()
        n193 = local write "Speed Antrieb"(w229) -> ()
        n194 = local write "Drehmoment Antrieb"(w256) -> ()
        n195 = local write "Status/Fehler Antrieb"(w257) -> ()
        n196 = local write "Digital Antrieb"(w255) -> ()
        n197 = Index Array(array=w295, index=15) -> (element=w254:bool)
        n198 = Index Array(array=w295, index=13) -> (element=w252:bool)
        n199 = Index Array(array=w295, index=14) -> (element=w253:bool)
        n200 = Index Array(array=w295, index=11) -> (element=w250:bool)
        n201 = Index Array(array=w295, index=12) -> (element=w251:bool)
        n202 = Index Array(array=w295, index=10) -> (element=w249:bool)
        n203 = Index Array(array=w295, index=9) -> (element=w248:bool)
        n204 = Index Array(array=w295, index=7) -> (element=w246:bool)
        n205 = Index Array(array=w295, index=8) -> (element=w247:bool)
        n206 = Index Array(array=w295, index=6) -> (element=w245:bool)
        n207 = Index Array(array=w295, index=5) -> (element=w244:bool)
        n208 = local write "Reserviert 8"(w252) -> ()
        n209 = local write "Standby aktiv 2"(w253) -> ()
        n210 = local write "Geschwindigkeit erreicht 2"(w250) -> ()
        n211 = local write "Warnung 2"(w248) -> ()
        n212 = local write "AS2 aktiv 2"(w249) -> ()
        n213 = local write "SWES inaktiv 2"(w251) -> ()
        n214 = local write "Handshake 3"(w254) -> ()
        n215 = Index Array(array=w295, index=3) -> (element=w242:bool)
        n216 = local write "in Position 2"(w246) -> ()
        n217 = local write "Fehler 2"(w247) -> ()
        n218 = Index Array(array=w295, index=1) -> (element=w240:bool)
        n219 = Index Array(array=w295, index=2) -> (element=w241:bool)
        n220 = Index Array(array=w295, index=4) -> (element=w243:bool)
        n221 = Index Array(array=w295, index=0) -> (element=w239:bool)
        n222 = local write "Relativposition übernommen 2"(w245) -> ()
        n223 = local write "referenziert 2"(w244) -> ()
        n224 = local write "Endstufenfreigabe 2"(w241) -> ()
        n225 = local write "Motor dreht 2"(w243) -> ()
        n226 = local write "Bremse geöffnet 2"(w242) -> ()
        n227 = local write "Betriebsbereit 2"(w239) -> ()
        n228 = local write "STO inaktiv 2"(w240) -> ()
      }
    }
    n229 = local read "VI-Stopp"() -> (w143:bool)
  }
  n230 = while {
    shift-right: [w330] -> w8
    shift-left: w6 -> [w328]
    shift-right: [w324] -> w9
    shift-left: w5 -> [w327]
    shift-right: [w329] -> w7
    shift-left: w4 -> [w326]
    stop <- w320 stop-if-true
    n231 = local read "Messung"() -> (w325:bool)
    n232 = case shown="False" w325 {
      tunnel: [w339 w477] -> w330
      tunnel: [w338 w475] -> w329
      tunnel: w328 -> [w337 w477]
      tunnel: w327 -> [w336 w476]
      tunnel: w326 -> [w335 w475]
      tunnel: [w340 w476] -> w324
      frame False {
        n233 = call <vilib>:"Is Path and Not Empty.vi"("path"="Datei-Pfad") -> ("Is Path and Not Empty?"=w333:bool)  [unwired: 4 in]
        n234 = case shown="True" w333 {
          tunnel: [w342 w404] -> w340
          tunnel: [w343 w403] -> w339
          tunnel: [w341 w402] -> w338
          tunnel: w337 -> [w346 w401]
          tunnel: w336 -> [w345 w400]
          tunnel: w335 -> [w344 w399]
          tunnel: "Datei-Pfad" -> [_ w395]
          frame False {
            # "Run data acquisition untill stop. DAQ-loop: Update signals and do anything with the  measurement values.\n(Here: show first signal in diagram)"
            n235 = while {
              tunnel: [w374] -> w342
              tunnel: [w373] -> w343
              tunnel: [w366] -> w341
              tunnel: w346 -> [w371]
              tunnel: w345 -> [w370]
              tunnel: w344 -> [w369]
              stop <- w352 stop-if-true
              n236 = call <userlib>:"UpdateMeasurementValues.vi"("Error in"=w369, "DaqMeasurement"=w370, "DevicesAndSignals"=w371) -> ("Error out"=w364:errorcluster, "DaqMeasurement"=w363:refnum<k24>, "DevicesAndSignals"=w365:T1)  [unwired: 6 in]
              n237 = local read "Kanal 2"() -> (w356:i32)
              n238 = local read "Kanal"() -> (w359:i32)
              n239 = Subtract(x=w359, y=1) -> (x-y=w358:i32)
              n240 = Subtract(x=w356, y=1) -> (x-y=w355:i32)
              n241 = call <userlib>:"GetMeasurementValues.vi"("Error in"=w364, "Index"=w358, "DaqMeasurement"=w363, "DevicesAndSignals"=w365) -> ("Error out"=w366:errorcluster, "Waveform"=w368:waveform(dbl), "DaqMeasurement"=w374:refnum<k24>, "DevicesAndSignals"=w373:T1)  [unwired: 2 in, 2 out]
              n242 = call <userlib>:"GetMeasurementValues.vi"("Error in"=w364, "Index"=w355, "DaqMeasurement"=w363, "DevicesAndSignals"=w365) -> ("Error out"=w362:errorcluster, "Waveform"=w361:waveform(dbl))  [unwired: 2 in, 4 out]
              n243 = local write "Diagram"(w368) -> ()
              n244 = local write "Diagram 2"(w361) -> ()
              n245 = local read "Messung"() -> (w353:bool)
              n246 = local read "VI-Stopp"() -> (w349:bool)
              n247 = local read "Numeric"() -> (w347:i32)
              n248 = Less?(x=w347, y=1) -> (x < y?=w350:bool)
              n249 = Or(x=w366, y=w362) -> (x .or. y?=w367:bool)
              n250 = Or(x=w353, y=w349) -> (x .or. y?=w354:bool)
              n251 = And(x=w349, y=w350) -> (x .and. y?=w348:bool)
              n252 = Or(x=w367, y=w354) -> (x .or. y?=w352:bool)
              n253 = case shown="True" w348 {
                frame False {
                }
                frame True {
                  n254 = local read "VI wird beendet"() -> (w376:string)
                  n255 = local write "Numeric"(1 ("Numeric")) -> ()
                  n256 = One Button Dialog(message=w376) -> ()  [unwired: 1 in, 1 out]
                }
              }
              n257 = Wait Until Next ms Multiple(millisecond multiple=u32 20 ("Vielfache von ms")) -> ()  [unwired: 1 out]
            }
          }
          frame True {
            # "Close\nFile"
            # "Create file path and file name"
            # "Run data acquisition until stop. DAQ-loop: Update signals and do anything with the  measurement values.\n(Here: show first signal in diagram + speichern der Daten in einer .txt file)"
            n258 = local read "Kanal 2"() -> (w388:i32)
            n259 = local read "Kanal"() -> (w389:i32)
            n260 = Not Equal?(x=w389, y=w388) -> (x != y?=w390:bool)
            n261 = case shown="True" w390 {
              tunnel: w395 -> [w423 w437]
              tunnel: [w407 w425] -> w392
              frame False {
                (unwired) i16 0 ("precision (6)")
                n262 = local read "Kanal"() -> (w421:i32)
                n263 = Add(x=w421, y=1) -> (x+y=w422:i32)
                n264 = call "ZeitabhängigeTXTerstellen.vi"("Signal index to display"=w422, "path"=w423) -> ("Path"=w419:path)  [unwired: 9 in]
                n265 = local read "Kanal 2"() -> (w408:i32)
                n266 = Open/Create/Replace File(file path (use dialog)=w419, operation (0:open)=T2."open or create", access (0:read/write)=enum16{"read/write", "read-only", "write-only"}."write-only") -> (refnum out=w409:refnum<file>)  [unwired: 3 in, 2 out]
                n267 = Get Date/Time String() -> (date string=w415:string)  [unwired: 3 in, 1 out]
                n268 = Number To Fractional String(number=w408, width (-)=i16 1) -> (F-format string=w411:string)  [unwired: 2 in]
                n269 = Concatenate Strings("Messung von " ("text"), w415, " Kanal " ("string"), w411, "\r\n") -> (w414:string)
                n270 = Write to Text File(file (use dialog)=w409, text=w414) -> (refnum out=w407:refnum<file>)  [unwired: 2 in, 2 out]
              }
              frame True {
                n271 = local read "Kanal 2"() -> (w439:i32)
                n272 = local read "Kanal 2"() -> (w427:i32)
                n273 = call "ZeitabhängigeTXTerstellen.vi"("Signal index to display"=w439, "path"=w437) -> ("Path"=w438:path)  [unwired: 9 in]
                n274 = Get Date/Time String() -> (date string=w433:string)  [unwired: 3 in, 1 out]
                n275 = Open/Create/Replace File(file path (use dialog)=w438, operation (0:open)=T2."open or create", access (0:read/write)=enum16{"read/write", "read-only", "write-only"}."write-only") -> (refnum out=w426:refnum<file>)  [unwired: 3 in, 2 out]
                n276 = Number To Fractional String(number=w427, width (-)=i16 1, precision (6)=i16 0) -> (F-format string=w429:string)  [unwired: 1 in]
                n277 = Concatenate Strings("Messung von " ("text"), w433, " Kanal " ("string"), w429, "\r\n") -> (w432:string)
                n278 = Write to Text File(file (use dialog)=w426, text=w432) -> (refnum out=w425:refnum<file>)  [unwired: 2 in, 2 out]
              }
            }
            n279 = local read "Kanal"() -> (w396:i32)
            n280 = local read "Kanal"() -> (w379:i32)
            n281 = call "ZeitabhängigeTXTerstellen.vi"("Signal index to display"=w396, "path"=w395) -> ("Path"=w391:path)  [unwired: 9 in]
            n282 = Get Date/Time String() -> (date string=w386:string)  [unwired: 3 in, 1 out]
            n283 = Number To Fractional String(number=w379, width (-)=i16 1, precision (6)=i16 0) -> (F-format string=w380:string)  [unwired: 1 in]
            n284 = Open/Create/Replace File(file path (use dialog)=w391, operation (0:open)=T2."open or create", access (0:read/write)=enum16{"read/write", "read-only", "write-only"}."write-only") -> (refnum out=w377:refnum<file>)  [unwired: 3 in, 2 out]
            n285 = Concatenate Strings("Messung von " ("text"), w386, " Kanal " ("string"), w380, "\r\n") -> (w385:string)
            n286 = Write to Text File(file (use dialog)=w377, text=w385) -> (refnum out=w384:refnum<file>)  [unwired: 2 in, 2 out]
            n287 = while {
              tunnel: w400 -> [w471]
              tunnel: [w470] -> w404
              tunnel: [w469] -> w403
              tunnel: w399 -> [w472]
              tunnel: [w456] -> w402
              tunnel: [w466] -> w406
              tunnel: [w465] -> w405
              tunnel: w384 -> [w464]
              tunnel: w401 -> [w463]
              tunnel: w392 -> [w458]
              tunnel: [w461] -> w398
              tunnel: [w460] -> w397
              stop <- w467 stop-if-true
              n288 = local read "Kanal 2"() -> (w448:i32)
              n289 = call <userlib>:"UpdateMeasurementValues.vi"("Error in"=w472, "DaqMeasurement"=w471, "DevicesAndSignals"=w463) -> ("Error out"=w455:errorcluster, "DaqMeasurement"=w453:refnum<k24>, "DevicesAndSignals"=w459:T1)  [unwired: 6 in]
              n290 = local read "Kanal"() -> (w452:i32)
              n291 = Subtract(x=w452, y=1) -> (x-y=w450:i32)
              n292 = Subtract(x=w448, y=1) -> (x-y=w447:i32)
              n293 = call <userlib>:"GetMeasurementValues.vi"("Error in"=w455, "Index"=w450, "DaqMeasurement"=w453, "DevicesAndSignals"=w459) -> ("Error out"=w456:errorcluster, "Waveform"=w462:waveform(dbl), "DaqMeasurement"=w470:refnum<k24>, "DevicesAndSignals"=w469:T1)  [unwired: 2 in, 2 out]
              n294 = call <userlib>:"GetMeasurementValues.vi"("Error in"=w455, "Index"=w447, "DaqMeasurement"=w453, "DevicesAndSignals"=w459) -> ("Waveform"=w457:waveform(dbl))  [unwired: 2 in, 5 out]
              n295 = local write "Diagram"(w462) -> ()
              n296 = call "MessdatenSchreiben.vi"("Waveform"=w462, "Byte Stream File in"=w464) -> ("error out"=w466:errorcluster, "Byte Stream File out"=w465:refnum<file>)  [unwired: 8 in]
              n297 = local read "Numeric"() -> (w440:i32)
              n298 = call "MessdatenSchreiben.vi"("Waveform"=w457, "Byte Stream File in"=w458) -> ("error out"=w460:errorcluster, "Byte Stream File out"=w461:refnum<file>)  [unwired: 8 in]
              n299 = local write "Diagram 2"(w457) -> ()
              n300 = local read "VI-Stopp"() -> (w442:bool)
              n301 = local read "Messung"() -> (w445:bool)
              n302 = Less?(x=w440, y=1) -> (x < y?=w443:bool)
              n303 = Or(x=w456, y=w455) -> (x .or. y?=w454:bool)
              n304 = And(x=w442, y=w443) -> (x .and. y?=w441:bool)
              n305 = Or(x=w445, y=w442) -> (x .or. y?=w446:bool)
              n306 = Wait Until Next ms Multiple(millisecond multiple=u32 20 ("Vielfache von ms")) -> ()  [unwired: 1 out]
              n307 = case shown="True" w441 {
                frame False {
                }
                frame True {
                  n308 = local read "VI wird beendet"() -> (w474:string)
                  n309 = local write "Numeric"(1 ("Numeric")) -> ()
                  n310 = One Button Dialog(message=w474) -> ()  [unwired: 1 in, 1 out]
                }
              }
              n311 = Or(x=w454, y=w446) -> (x .or. y?=w467:bool)
            }
            n312 = Close File(refnum=w398, error in=w397) -> ()  [unwired: 2 out]
            n313 = Close File(refnum=w405, error in=w406) -> ()  [unwired: 2 out]
          }
        }
      }
      frame True {
        n314 = while {
          stop <- w483 stop-if-true
          n315 = Wait (ms)(milliseconds to wait=u32 10) -> ()  [unwired: 1 out]
          n316 = local read "Numeric"() -> (w480:i32)
          n317 = local read "Messung"() -> (w484:bool)
          n318 = local read "VI-Stopp"() -> (w481:bool)
          n319 = Less?(x=w480, y=1) -> (x < y?=w478:bool)
          n320 = And(x=w481, y=w478) -> (x .and. y?=w482:bool)
          n321 = Or(x=w484, y=w481) -> (x .or. y?=w483:bool)
          n322 = case shown="True" w482 {
            frame False {
            }
            frame True {
              n323 = local read "VI wird beendet"() -> (w487:string)
              n324 = local write "Numeric"(1 ("Numeric")) -> ()
              n325 = One Button Dialog(message=w487) -> ()  [unwired: 1 in, 1 out]
            }
          }
        }
      }
    }
    n326 = local read "VI-Stopp"() -> (w320:bool)
    n327 = local read "Numeric"() -> (w319:i32)
    n328 = Less?(x=w319, y=1) -> (x < y?=w323:bool)
    n329 = And(x=w320, y=w323) -> (x .and. y?=w321:bool)
    n330 = case shown="True" w321 {
      frame False {
      }
      frame True {
        n331 = local read "VI wird beendet"() -> (w332:string)
        n332 = local write "Numeric"(1 ("Numeric")) -> ()
        n333 = One Button Dialog(message=w332) -> ()  [unwired: 1 in, 1 out]
      }
    }
  }
  n334 = call <userlib>:"StopDaq.vi"("Error in"=w7, "DaqMeasurement"=w9, "DevicesAndSignals"=w8) -> ("Error out"=w17:errorcluster, "DevicesAndSignals"=w16:T1)  [unwired: 7 in]
  n335 = call <userlib>:"DisconnectDevice.vi"("Error in"=w17, "DevicesAndSignals"=w16) -> ("Error out"=w15:errorcluster)  [unwired: 9 in]
  n336 = call <vilib>:"Simple Error Handler.vi"("error in (no error)"=w15) -> ("error out"=w34:errorcluster)  [unwired: 4 in, 4 out]
  n337 = call <userlib>:"DisposeApi.vi"("Error in"=w34) -> ()  [unwired: 10 in, 1 out]
  "VI wird beendet" <- "VI wird ordnungsgemäß beendet, bitte einen Moment Geduld"
  "Numeric" <- 0
  "N" <- -1
